vi "example_GArrayUpload.vi"() -> ()   [LabVIEW 2020]
uses:
  <vilib>/Galil/resources/gclib32/gclib32.lvlib
panel:
  out "Uploaded Array":string
  out "Response":string
  in  "Command":string="DM A[100]"
  out "Error Out":errorcluster
  in  "IP Address":string="192.168.1.77"
  in  "Downloaded Array":string="100,120,140,160,180,200"
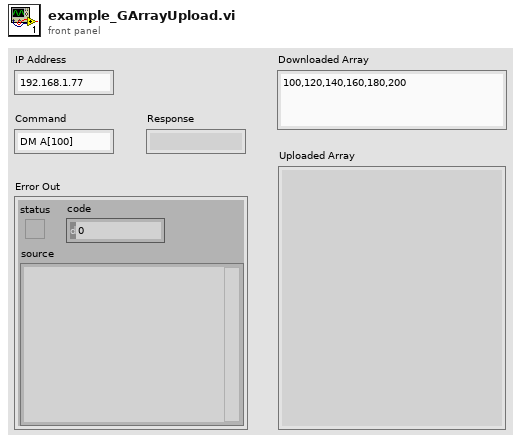
[diagram p1: front panel]
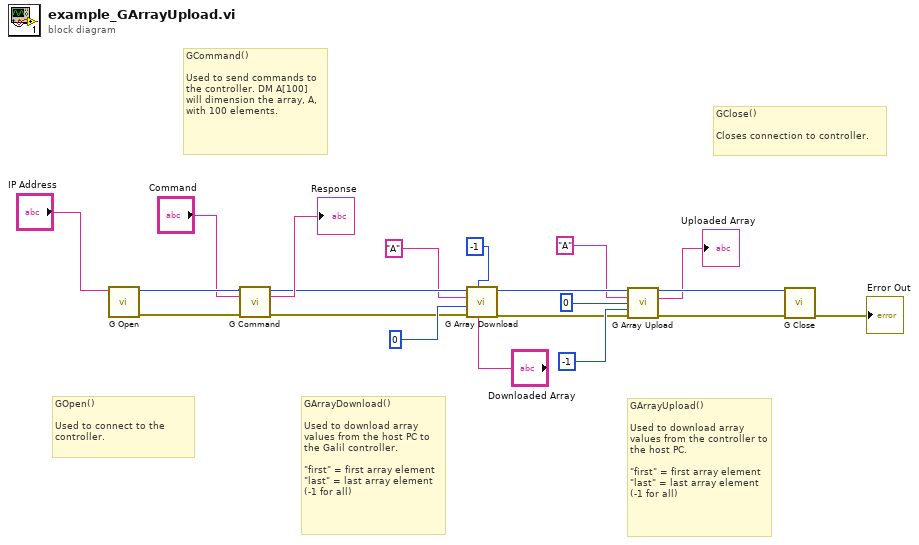
[diagram p0: block diagram]
diagram:
  # "GClose()\n\nCloses connection to controller."
  # "GArrayUpload()\n\nUsed to download array values from the controller to the host PC. \n\n\"first\" = first array element\n\"last\" = last array element (-1 for all)"
  # "GArrayDownload()\n\nUsed to download array values from the host PC to the Galil controller.\n\n\"first\" = first array element\n\"last\" = last array element (-1 for all)"
  # "GCommand()\n\nUsed to send commands to the controller. DM A[100] will dimension the array, A, with 100 elements."
  # "GOpen()\n\nUsed to connect to the controller."
  n1 = call <vilib>:"G Open.vi"("address"="IP Address") -> ("error out"=w18:errorcluster, "g out"=w17:u32)  [unwired: 8 in]
  n2 = call <vilib>:"G Command.vi"("g"=w17, "command"="Command", "error in (no error)"=w18) -> ("g out"=w14:u32, "buffer out"=→"Response":string, "error out"=w11:errorcluster)  [unwired: 10 in]
  n3 = call <vilib>:"G Array Download.vi"("buffer"="Downloaded Array", "last"=-1, "error in (no error)"=w11, "first"=0, "array_name"="A", "g"=w14) -> ("error out"=w3:errorcluster, "g out"=w8:u32)  [unwired: 4 in]
  n4 = call <vilib>:"G Array Upload.vi"("g"=w8, "array_name"="A", "first"=0, "last"=-1, "error in (no error)"=w3) -> ("g out"=w2:u32, "buffer out"=→"Uploaded Array":string, "error out"=w4:errorcluster)  [unwired: 8 in]
  n5 = call <vilib>:"G Close.vi"("error in (no error)"=w4, "g"=w2) -> ("error out"=→"Error Out":errorcluster)  [unwired: 9 in]
